vi "LinearSystemId_CreateElevatorSystem.vi"(8 "G":dbl, 9 "radiusMeters":dbl, 10 "massKg":dbl, 11 "DCMOTOR":T1 {"Jr_KgM2" format="%13.5p"; "L_H" format="%13.5p"; "Kt_NMPerAmp" format="%13.5p"; "KvINV_RadPerSecPerVolt" format="%13.5p"; "R_Ohms" format="%13.5p"; "FreeSpeed_RadPerSec" format="%13.5p"; "FreeCurrent_Amps" format="%13.5p"; "StallCurrent_Amps" format="%13.5p"; "StallTorque_NM" format="%13.5p"; "nominalVoltage_Volts" format="%13.5p"}) -> (0 "Size Coerced":bool, 3 "Linearsystem":T2)   [LabVIEW 2019, in "Trajectory_Library.lvlib"]
doc: "Create a state-space model of an elevator system. The states of the system are [position, velocity]?, inputs are [voltage], and outputs are [position].\n\nInputs: \n - motor -- The motor (or gearbox) attached to the arm.\n - massKg -- The mass of the elevator carriage, in kilograms.\n - radiusMeters -- The radius of thd driving drum of the elevator, in meters.\n - G -- The reduction between motor and drum, as a ratio of output to input.\n\nOutputs:\n - LinearSystem -- A LinearSystem representing the given characterized constants.\n - SizeCoerced -- A boolean indicating that sizes had to be adjusted. A value of TRUE indicates an error."
uses:
  Trajectory_Library.lvlib
  LINEAR_SYSTEM.ctl
  <vilib>/Analysis/Matrix/Datatypes/RealMatrix.ctl
  DCMOTOR.CTL
  <vilib>/Analysis/Matrix/NI_Matrix.lvlib
panel:
  # "<States,States>"
  # "<States,Inputs>"
  # "<Outputs,States>"
  # "<Outputs,Inputs>"
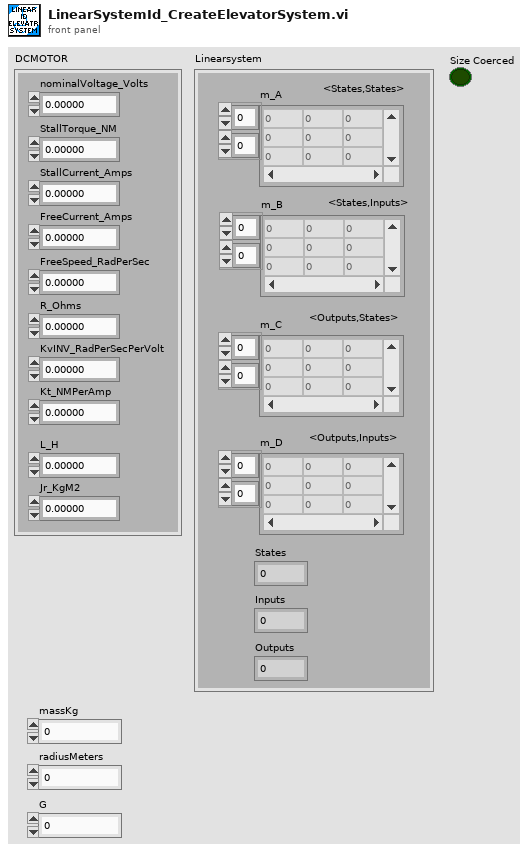
[diagram p1: front panel]
types:
  T1 = typedef "Trajectory_Library.lvlib/DCMOTOR.CTL" = cluster{"nominalVoltage_Volts":dbl, "StallTorque_NM":dbl, "StallCurrent_Amps":dbl, "FreeCurrent_Amps":dbl, "FreeSpeed_RadPerSec":dbl, "R_Ohms":dbl, "KvINV_RadPerSecPerVolt":dbl, "Kt_NMPerAmp":dbl, "L_H":dbl, "Jr_KgM2":dbl}
  T2 = typedef "Trajectory_Library.lvlib/LINEAR_SYSTEM.ctl" = cluster{"m_A":T3, "m_B":T3, "m_C":T3, "m_D":T3, "States":i32, "Inputs":i32, "Outputs":i32}
  T3 = typedef "NI_Matrix.lvlib/RealMatrix.ctl" = dbl[][]
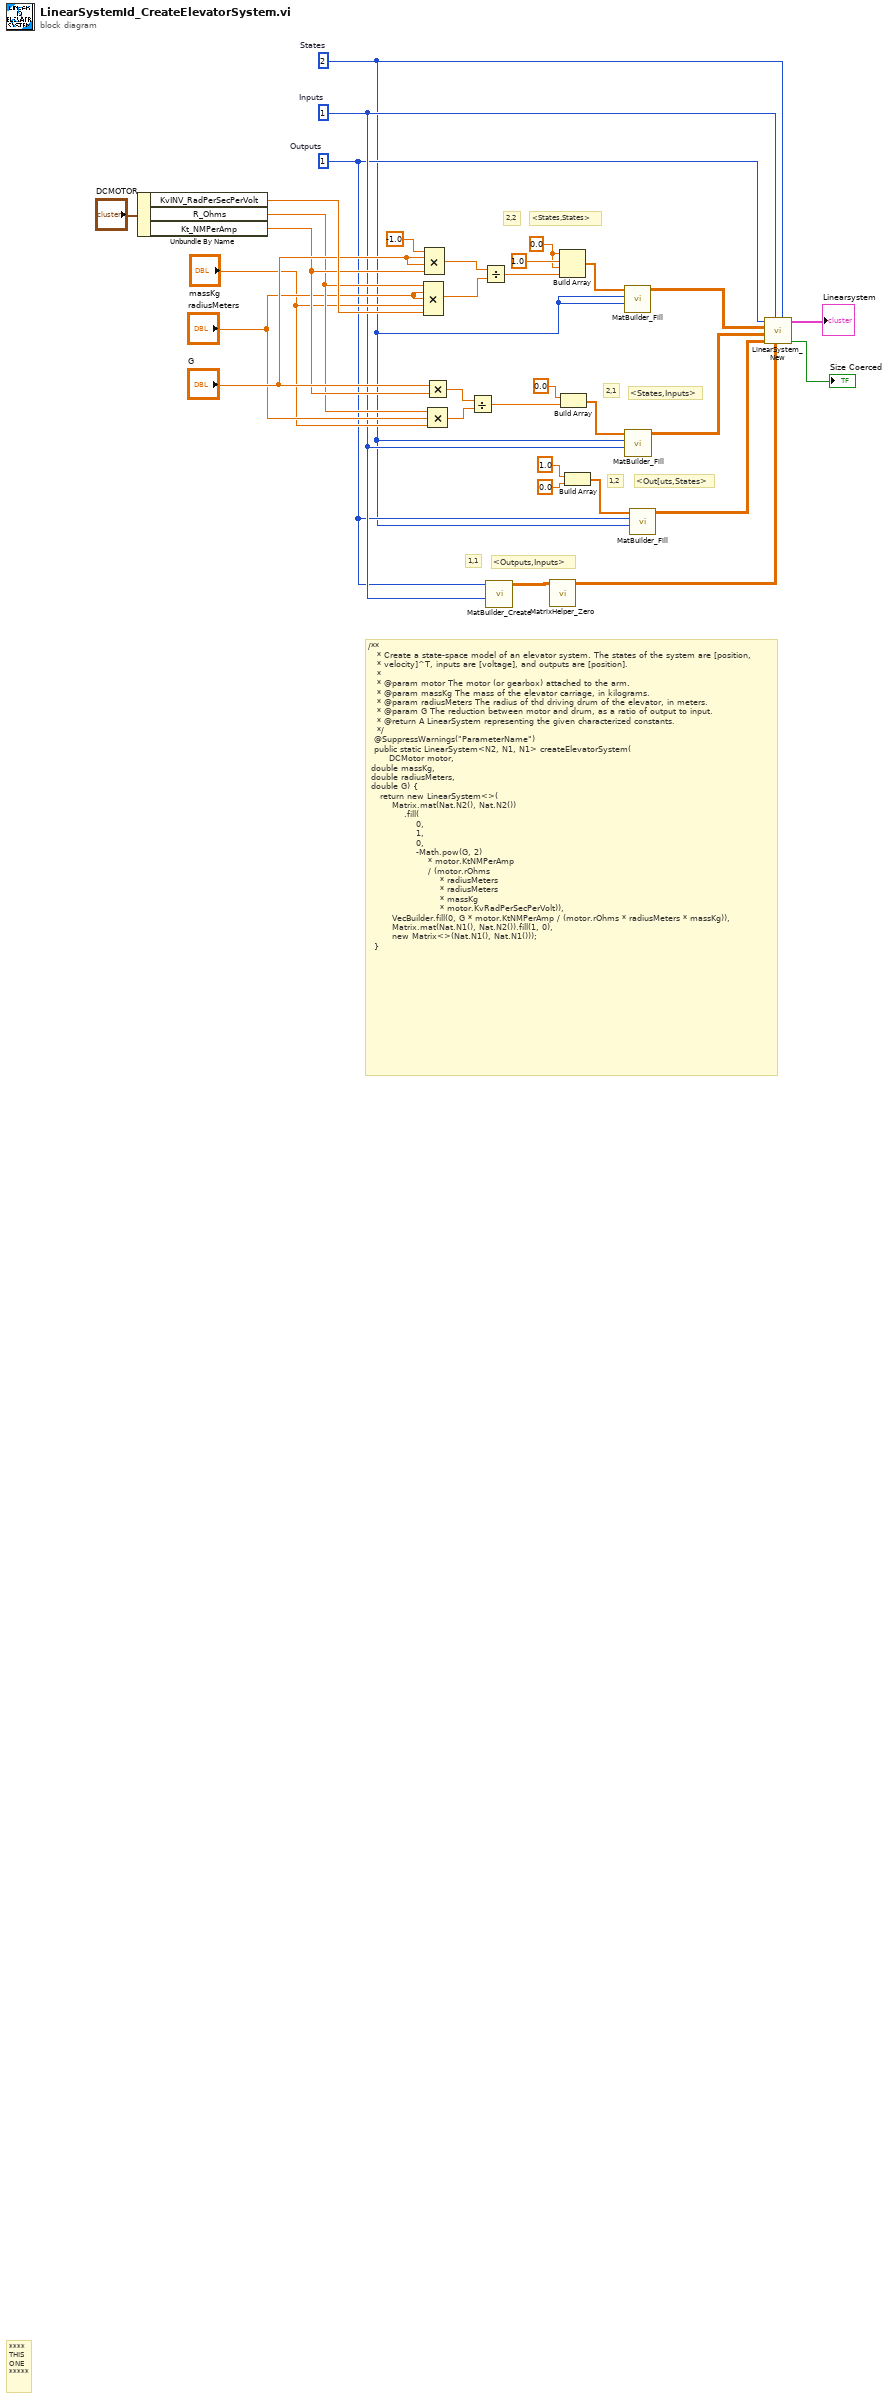
[diagram p0: block diagram]
diagram:
  w10 = 1  # Outputs
  w18 = 1  # Inputs
  w2 = 2  # States
  w5 = 0.0 ("element")
  # "2,2"
  # "2,1"
  # "1,2"
  # "1,1"
  # "<States,States>"
  # "<States,Inputs>"
  # "<Out[uts,States>"
  # "<Outputs,Inputs>"
  # "/**\n   * Create a state-space model of an elevator system. The states of the system are [position,\n   * velocity]^T, inputs are [voltage], and outputs are [position].\n   *\n   * @param motor The motor (or gearbox) attached to the arm.\n   * @param massKg The mass of the elevator carriage, in kilograms.\n   * @param radiusMeters The radius of thd driving drum of the elevator, in meters.\n   * @param G The reduction between motor and drum, as a ratio of output to input.\n   * @return A LinearSystem representing the given characterized constants.\n   */\n  @SuppressWarnings(\"ParameterName\")\n  public static LinearSystem<N2, N1, N1> createElevatorSystem(\n      \tDCMotor motor, \n\tdouble massKg, \n\tdouble radiusMeters, \n\tdouble G) {\n    return new LinearSystem<>(\n        Matrix.mat(Nat.N2(), Nat.N2())\n            .fill(\n                0,\n                1,\n                0,\n                -Math.pow(G, 2)\n                    * motor.KtNMPerAmp\n                    / (motor.rOhms\n                        * radiusMeters\n                        * radiusMeters\n                        * massKg\n                        * motor.KvRadPerSecPerVolt)),\n        VecBuilder.fill(0, G * motor.KtNMPerAmp / (motor.rOhms * radiusMeters * massKg)),\n        Matrix.mat(Nat.N1(), Nat.N2()).fill(1, 0),\n        new Matrix<>(Nat.N1(), Nat.N1()));\n  }"
  # "****\nTHIS\nONE\n*****"
  n1 = Unbundle By Name("DCMOTOR") -> ("KvINV_RadPerSecPerVolt"=w29:dbl, "R_Ohms"=w22:dbl, "Kt_NMPerAmp"=w25:dbl)
  n2 = Compound Arithmetic op=MULTIPLY(w22, "radiusMeters", "radiusMeters", "massKg", w29) -> (w27:dbl)
  n3 = Compound Arithmetic op=MULTIPLY(-1.0 ("value"), "G", "G", w25) -> (w28:dbl)
  n4 = Multiply(x="G", y=w25) -> (x*y=w24:dbl)
  n5 = Compound Arithmetic op=MULTIPLY(w22, "radiusMeters", "massKg") -> (w23:dbl)
  n6 = Divide(x=w24, y=w23) -> (x/y=w16:dbl)
  n7 = Divide(x=w28, y=w27) -> (x/y=w4:dbl)
  n8 = call "MatBuilder_Create.vi"("Columns"=w18, "Rows"=w10) -> ("output matrix"=w9:T3)  [unwired: 9 in]
  n9 = call "MatrixHelper_Zero.vi"("input matrix"=w9) -> ("output matrix"=w8:T3)  [unwired: 10 in]
  n10 = Build Array(w5, 1.0 ("element"), w5, w4) -> (w7:dbl[])
  n11 = Build Array(0.0 ("element"), w16) -> (w19:dbl[])
  n12 = Build Array(1.0 ("element"), 0.0 ("element")) -> (w14:dbl[])
  n13 = call "MatBuilder_Fill.vi"("Columns"=w2, "Rows"=w2, "Value List"=w7) -> ("output matrix"=w3:T3)  [unwired: 8 in]
  n14 = call "MatBuilder_Fill.vi"("Columns"=w18, "Rows"=w2, "Value List"=w19) -> ("output matrix"=w15:T3)  [unwired: 8 in]
  n15 = call "MatBuilder_Fill.vi"("Columns"=w2, "Rows"=w10, "Value List"=w14) -> ("output matrix"=w12:T3)  [unwired: 8 in]
  n16 = call "LinearSystem_New.vi"("States"=w2, "D"=w8, "Inputs"=w18, "C"=w12, "B"=w15, "A"=w3, "Outputs"=w10) -> ("Size Coerced"=→"Size Coerced":bool, "Linearsystem"=→"Linearsystem":T2)  [unwired: 3 in]
